vi "Calculate Indent.vi"(1 "input":string[](array[string])) -> (0 "indent":i32[](array[numeric]))   [LabVIEW 2017, in "Error File Management.lvlib"]
uses:
  Error File Management.lvlib
  <vilib>/regexp/Match Regular Expression.xnode
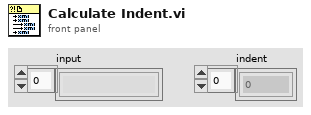
[diagram p1: front panel]
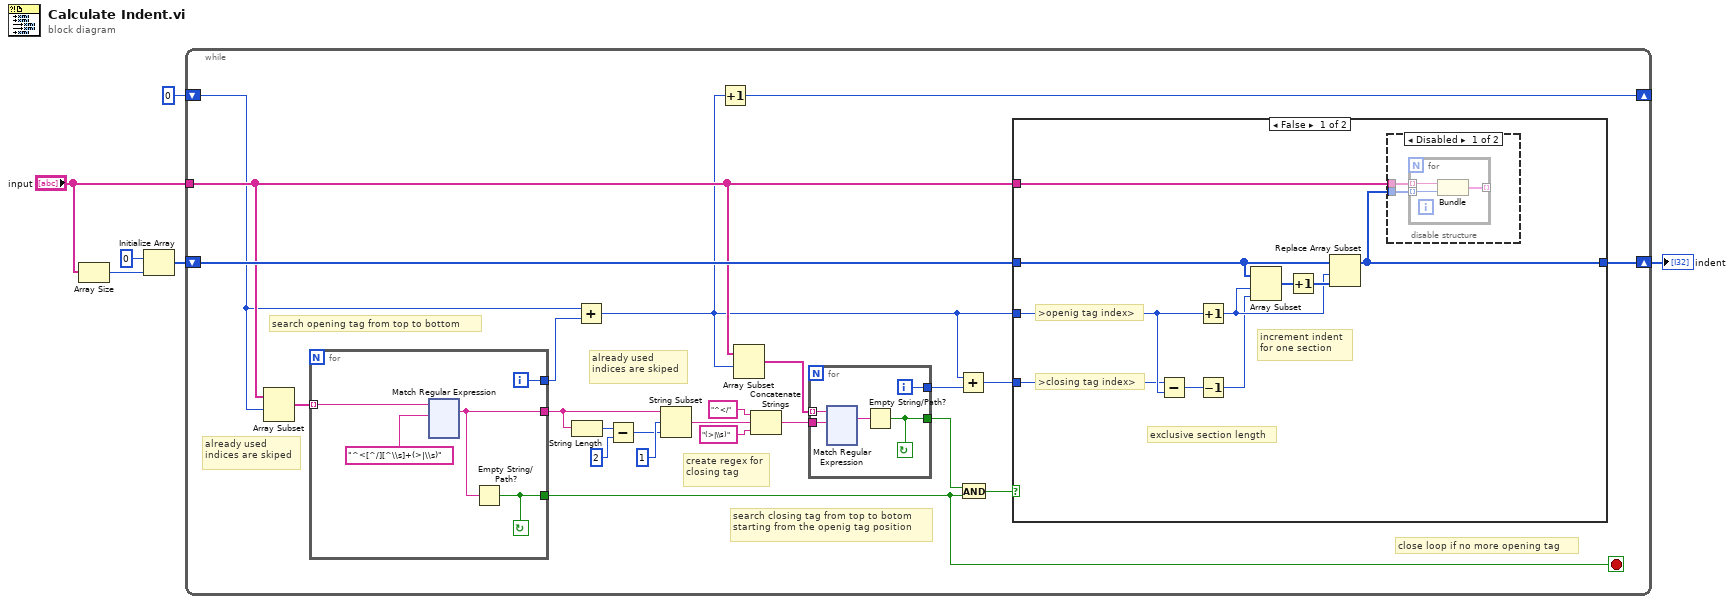
[diagram p0: block diagram]
diagram:
  n1 = Array Size(array="input") -> (size(s)=w5:i32)
  n2 = Initialize Array(0 ("x-y"), w5) -> (w6:i32[])
  n3 = while {
    shift-right: [w21] -> w2
    shift-left: w6 -> [w23]
    tunnel: "input" -> [w12]
    shift-right: [w13] -> _
    shift-left: 0 ("x-y") -> [w10]
    stop <- w17 stop-if-true
    # "search closing tag from top to botom starting from the openig tag position"
    # "create regex for closing tag"
    # "search opening tag from top to bottom"
    # "close loop if no more opening tag"
    # "already used indices are skiped"
    # "already used indices are skiped"
    n4 = Array Subset(array=w12, index=w10) -> (w16:string[])  [unwired: 1 in]
    n5 = for {
      tunnel: w16 -> [w34] mode=indexing
      tunnel: [w31] -> w15
      tunnel: [w33] -> w17
      tunnel: [w32] -> w28
      i -> [w31]
      stop <- w33 continue-if-true
      n6 = xnode "Match Regular Expression"("input string"=w34, "regular expression"="^<[^/][^\\s]+(>|\\s)") -> ("whole match"=w32:string)  [unwired: 4 in, 4 out]
      n7 = Empty String/Path?(string/path=w32) -> (empty?=w33:bool)
    }
    n8 = String Length(string=w28) -> (length=w27:i32)
    n9 = Add(x=w10, y=w15) -> (x+y=w7:i32)
    n10 = Subtract(x=w27, y=2 ("x")) -> (x-y=w20:i32)
    n11 = String Subset(string=w28, offset (0)=1, length (rest)=w20) -> (substring=w26:string)
    n12 = Increment(x=w7) -> (x+1=w13:i32)
    n13 = Array Subset(array=w12, index=w7) -> (w11:string[])  [unwired: 1 in]
    n14 = Concatenate Strings("^</" ("string"), w26, "(>|\\s)" ("string")) -> (w14:string)
    n15 = for {
      tunnel: w11 -> [w153] mode=indexing
      tunnel: [w152] -> w9
      tunnel: [w149] -> w22
      tunnel: w14 -> [w150]
      i -> [w152]
      stop <- w149 continue-if-true
      n16 = xnode "Match Regular Expression"("input string"=w153, "regular expression"=w150) -> ("whole match"=w151:string)  [unwired: 4 in, 4 out]
      n17 = Empty String/Path?(string/path=w151) -> (empty?=w149:bool)
    }
    n18 = Add(x=w7, y=w9) -> (x+y=w8:i32)
    n19 = And(x=w22, y=w17) -> (x .and. y?=w18:bool)
    n20 = case shown="False" w18 {
      tunnel: w23 -> [w276 w283]
      tunnel: w7 -> [w272 _]
      tunnel: [w270 w283] -> w21
      tunnel: w12 -> [w271 _]
      tunnel: w8 -> [w269 _]
      frame False {
        # "exclusive section length"
        # ">closing tag index>"
        # ">openig tag index>"
        # "increment indent for one section"
        n21 = Subtract(x=w269, y=w272) -> (x-y=w268:i32)
        n22 = Increment(x=w272) -> (x+1=w274:i32)
        n23 = Decrement(x=w268) -> (x-1=w273:i32)
        n24 = Array Subset(array=w276, index=w274, length=w273) -> (w277:i32[])
        n25 = Increment(x=w277) -> (x+1=w275:i32[])
        n26 = Replace Array Subset(array=w276, new element=w275, index=w274) -> (w270:i32[])
        n27 = disable-structure shown="Disabled" {
          disable-tunnel: w271 -> [w279 _]
          disable-tunnel: w270 -> [w278 _]
          frame Disabled {
            n28 = for {
              tunnel: w279 -> [w282] mode=indexing
              tunnel: w278 -> [w281] mode=indexing
              tunnel: [w280] -> _ mode=indexing
              n29 = Bundle("trimmed string"=w282, "x-y"=w281) -> (w280:cluster{"trimmed string":string, "x-y":i32})  [unwired: 1 in]
            }
          }
          frame Enabled {
          }
        }
      }
      frame True {
      }
    }
  }
  "indent" <- w2
